vi "Post-Build Action.vi"(5 "Files Generated by Build":path[](array[path]), 6 "Top Level/Always Included VIs":path[](array[path]), 7 "Destination Path":path, 8 "error in (no error)":errorcluster, 9 "Target Name":string, 10 "Build Specification Name":string, 11 "Project Path":path) -> (0 "error out":errorcluster)   [LabVIEW 2017]
doc: "This VI is called after each run of a build specification. The VI will copy the generated LLB (Engine or System Explorer) into the VeriStand Custom Device folder (...\\Documents\\National Instruments\\NI VeriStand 2013...)."
uses:
  <vilib>/Utility/sysdir.llb/System Directory Type.ctl
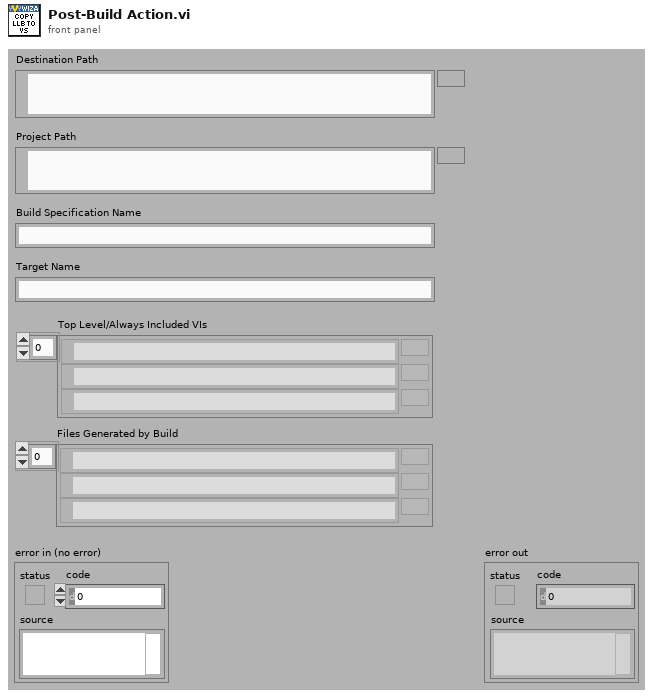
[diagram p1: front panel]
types:
  T1 = typedef "System Directory Type.ctl" = i32
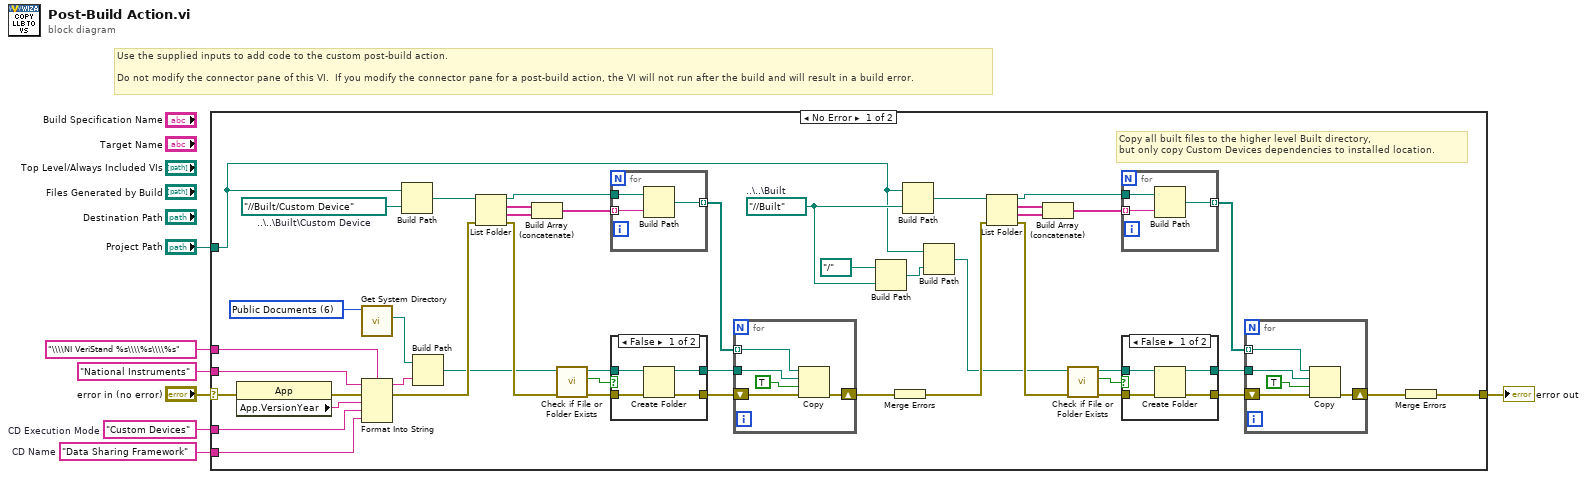
[diagram p0: block diagram]
diagram:
  w2 = "Data Sharing Framework"  # CD Name
  w3 = "Custom Devices"  # CD Execution Mode
  # "Use the supplied inputs to add code to the custom post-build action.\n\nDo not modify the connector pane of this VI.  If you modify the connector pane for a post-build action, the VI will not run after the build and will result in a build error."
  n1 = case shown="No Error" "error in (no error)" {
    selector: "error in (no error)" -> [w36 w82]
    tunnel: [w24 w82] -> w5
    tunnel: "Project Path" -> [w18 _]
    tunnel: "\\\\NI VeriStand %s\\\\%s\\\\%s" ("name or relative path") -> [w39 _]
    tunnel: w3 -> [w38 _]
    tunnel: w2 -> [w37 _]
    tunnel: "National Instruments" ("name or relative path") -> [w33 _]
    frame No Error {
      w20 = path "../../Built"  # ..\..\Built
      w32 = path "../../Built/Custom Device"  # ..\..\Built\Custom Device
      w42 = T1 6 items=["User Home"=0, "User Desktop"=1, "User Documents"=2, "User Application Data"=3, "User Preferences"=4, "User Temporary"=5, "Public Documents"=6, "Public Application Data"=7, "Public Preferences"=8, "Public Cache"=13, "System Core Libraries"=9, "System Installed Libraries"=10, "Application Files"=11, "Boot Volume Root"=12] ("system directory type")
      # "Copy all built files to the higher level Built directory,\nbut only copy Custom Devices dependencies to installed location."
      n2 = property class="App"(error in=w36) -> (error out=w41:errorcluster, "App.VersionYear"=w40:string)  [unwired: 1 in, 1 out]
      n3 = call <vilib>:"Get System Directory.vi"("system directory type"=w42) -> ("system directory"=w43:path)  [unwired: 10 in]
      n4 = Format Into String(format string=w39, initial string=w33, error in=w41, w40, w38, w37) -> (resulting string=w44:string, error out=w35:errorcluster)
      n5 = Build Path(base path=w18, name or relative path=w32) -> (appended path=w51:path)
      n6 = Build Path(base path=w43, name or relative path=w44) -> (appended path=w21:path)
      n7 = List Folder(path=w51, error in=w35) -> (path out=w53:path, filenames=w49:string[], folder names=w48:string[], error out=w52:errorcluster)  [unwired: 2 in]
      n8 = Build Array (concatenate)(w49, w48) -> (w47:string[])
      n9 = call <vilib>:"Check if File or Folder Exists.vi"("error in (no error)"=w52, "path"=w21) -> ("error out"=w15:errorcluster, "file or folder exists?"=w17:bool, "dup path"=w16:path)  [unwired: 7 in]
      n10 = for {
        tunnel: w47 -> [w80] mode=indexing
        tunnel: w53 -> [w81]
        tunnel: [w79] -> w34 mode=indexing
        n11 = Build Path(base path=w81, name or relative path=w80) -> (appended path=w79:path)
      }
      n12 = case shown="False" w17 {
        tunnel: w16 -> [w68 w70]
        tunnel: w15 -> [w67 w69]
        tunnel: [w66 w70] -> w14
        tunnel: [w65 w69] -> w13
        frame False {
          n13 = Create Folder(path (use dialog)=w68, error in=w67) -> (created path=w66:path, error out=w65:errorcluster)  [unwired: 1 in, 1 out]
        }
        frame True {
        }
      }
      n14 = for {
        tunnel: w34 -> [w72] mode=indexing
        shift-right: [w73] -> w50
        shift-left: w13 -> [w74]
        tunnel: w14 -> [w71]
        n15 = Copy(8:w74, 9:TRUE ("overwrite (F)"), 10:w71, 11:w72) -> (0:w73:errorcluster)  [unwired: 1 in, 2 out]
      }
      n16 = Build Path(base path=path "../..", name or relative path=w20) -> (appended path=w46:path)
      n17 = Merge Errors(w50) -> (w23:errorcluster)
      n18 = Build Path(base path=w18, name or relative path=w20) -> (appended path=w19:path)
      n19 = Build Path(base path=w18, name or relative path=w46) -> (appended path=w22:path)
      n20 = List Folder(path=w19, error in=w23) -> (path out=w25:path, filenames=w28:string[], folder names=w29:string[], error out=w26:errorcluster)  [unwired: 2 in]
      n21 = Build Array (concatenate)(w28, w29) -> (w30:string[])
      n22 = call <vilib>:"Check if File or Folder Exists.vi"("error in (no error)"=w26, "path"=w22) -> ("error out"=w10:errorcluster, "file or folder exists?"=w12:bool, "dup path"=w11:path)  [unwired: 7 in]
      n23 = for {
        tunnel: w30 -> [w77] mode=indexing
        tunnel: w25 -> [w78]
        tunnel: [w76] -> w31 mode=indexing
        n24 = Build Path(base path=w78, name or relative path=w77) -> (appended path=w76:path)
      }
      n25 = case shown="False" w12 {
        tunnel: w11 -> [w57 w59]
        tunnel: w10 -> [w56 w58]
        tunnel: [w55 w59] -> w9
        tunnel: [w54 w58] -> w8
        frame False {
          n26 = Create Folder(path (use dialog)=w57, error in=w56) -> (created path=w55:path, error out=w54:errorcluster)  [unwired: 1 in, 1 out]
        }
        frame True {
        }
      }
      n27 = for {
        tunnel: w31 -> [w61] mode=indexing
        shift-right: [w62] -> w27
        shift-left: w8 -> [w63]
        tunnel: w9 -> [w60]
        n28 = Copy(8:w63, 9:TRUE ("overwrite (F)"), 10:w60, 11:w61) -> (0:w62:errorcluster)  [unwired: 1 in, 2 out]
      }
      n29 = Merge Errors(w27) -> (w24:errorcluster)
    }
    frame Error {
    }
  }
  "error out" <- w5
